vi "AnalyzeBlobs.vi"(9 "Vision Target":enum16{"Pegs", "Gears"}(ring), 10 "Blob Data":T2, 11 "Image In":T3) -> (2 "Target Data":T1, 3 "Image Out":T3)   [LabVIEW 2016]
doc: "Returns if there is a target, and the angle and distance to the target"
uses:
  <vilib>/vision/Image Controls.llb/IMAQ Image.ctl
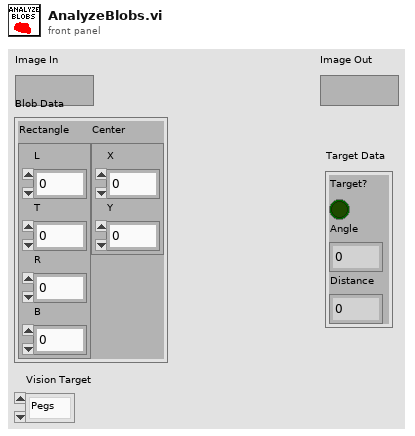
[diagram p1: front panel]
types:
  T1 = cluster{"Target?":bool, "Angle":dbl, "Distance":dbl}
  T2 = cluster{"Rectangle":cluster{"L":dbl, "T":dbl, "R":dbl, "B":dbl}, "Center":cluster{"X":dbl, "Y":dbl}}
  T3 = typedef "IMAQ Image.ctl" = refnum<image>
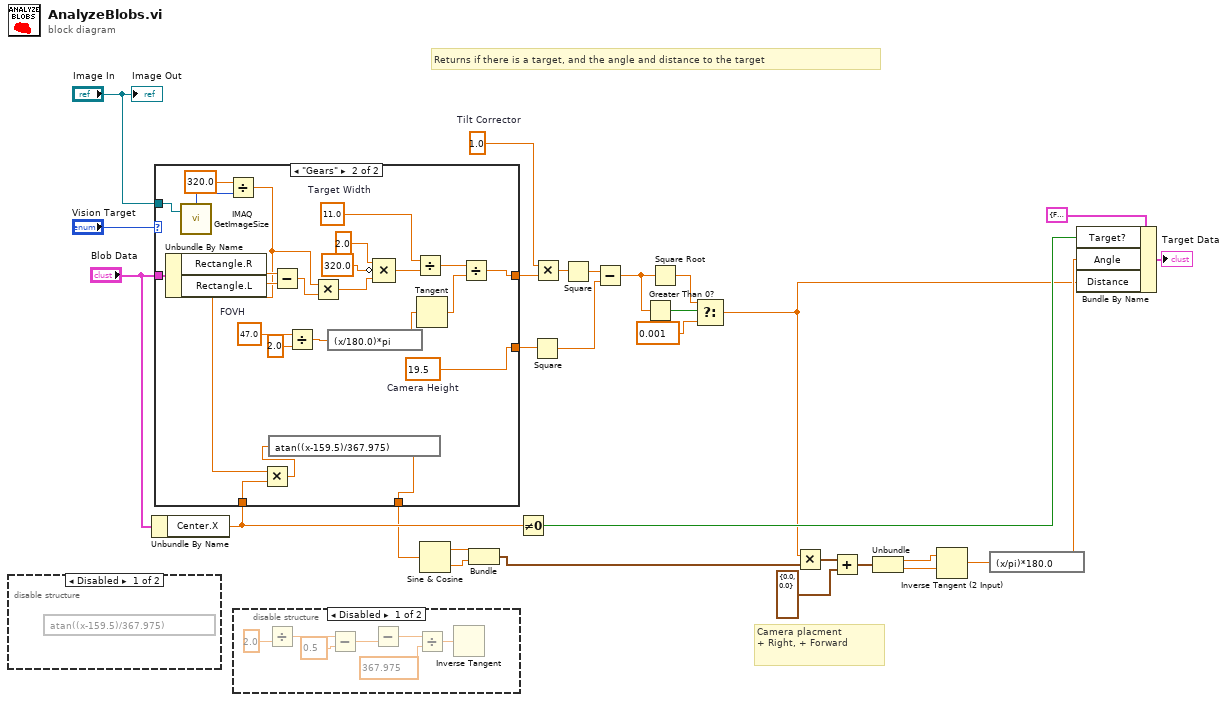
[diagram p0: block diagram]
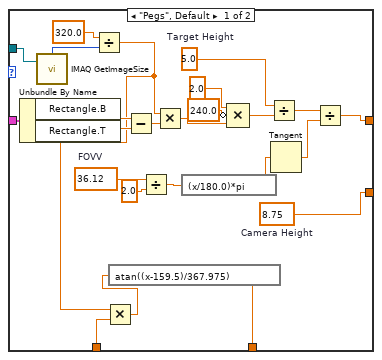
[diagram p4: hidden frame]
diagram:
  w28 = 1.0  # Tilt Corrector
  # "Returns if there is a target, and the angle and distance to the target"
  # "Camera placment\n+ Right, + Forward"
  n1 = disable-structure shown="Disabled" {
    frame Disabled {
      n2 = expression code="atan((x-159.5)/367.975)" ("degrees to radians")() -> ()  [unwired: 1 in, 1 out]
    }
    frame Enabled {
    }
  }
  n3 = Unbundle By Name("Blob Data") -> ("Center.X"=w2:dbl)
  n4 = case shown="\"Gears\"" "Vision Target" {
    tunnel: "Blob Data" -> [w53 w77]
    tunnel: [w44 w70] -> w27
    tunnel: [w43 w69] -> w25
    tunnel: "Image In" -> [w38 w64]
    tunnel: w2 -> [w32 w61]
    tunnel: [w37 w62] -> w1
    frame "Pegs", Default {
      w43 = 8.75  # Camera Height
      w49 = 36.12  # FOVV
      w40 = 5.0  # Target Height
      n5 = Unbundle By Name(w53) -> ("Rectangle.B"=w51:dbl, "Rectangle.T"=w52:dbl)
      n6 = call "IMAQ GetImageSize"("Image"=w38) -> ("X Resolution"=w35:i32)  [unwired: 3 in, 2 out]
      n7 = Divide(x=320.0 ("value"), y=w35) -> (x/y=w31:dbl)
      n8 = Multiply(x=w31, y=w32) -> (x*y=w30:dbl)
      n9 = expression code="atan((x-159.5)/367.975)" ("degrees to radians")(w30) -> (w37:dbl)
      n10 = Subtract(x=w51, y=w52) -> (x-y=w34:dbl)
      n11 = Divide(x=w49, y=2.0) -> (x/y=w47:dbl)
      n12 = Multiply(x=w31, y=w34) -> (x*y=w33:dbl)
      n13 = expression code="(x/180.0)*pi" ("degrees to radians")(w47) -> (w46:dbl)
      n14 = Compound Arithmetic op=MULTIPLY(2.0 ("value"), invert 240.0 ("value"), w33) -> (w41:dbl)
      n15 = Divide(x=w40, y=w41) -> (x/y=w39:dbl)
      n16 = Tangent(1:w46) -> (0:w45:dbl)
      n17 = Divide(x=w39, y=w45) -> (x/y=w44:dbl)
    }
    frame "Gears" {
      w69 = 19.5  # Camera Height
      w74 = 47.0  # FOVH
      w66 = 11.0  # Target Width
      n18 = Unbundle By Name(w77) -> ("Rectangle.R"=w75:dbl, "Rectangle.L"=w76:dbl)
      n19 = call "IMAQ GetImageSize"("Image"=w64) -> ("X Resolution"=w57:i32)  [unwired: 3 in, 2 out]
      n20 = Divide(x=320.0 ("value"), y=w57) -> (x/y=w55:dbl)
      n21 = Multiply(x=w55, y=w61) -> (x*y=w60:dbl)
      n22 = expression code="atan((x-159.5)/367.975)" ("degrees to radians")(w60) -> (w62:dbl)
      n23 = Subtract(x=w75, y=w76) -> (x-y=w56:dbl)
      n24 = Divide(x=w74, y=2.0) -> (x/y=w73:dbl)
      n25 = Multiply(x=w55, y=w56) -> (x*y=w54:dbl)
      n26 = expression code="(x/180.0)*pi" ("degrees to radians")(w73) -> (w72:dbl)
      n27 = Compound Arithmetic op=MULTIPLY(2.0 ("value"), invert 320.0 ("value"), w54) -> (w67:dbl)
      n28 = Divide(x=w66, y=w67) -> (x/y=w65:dbl)
      n29 = Tangent(1:w72) -> (0:w71:dbl)
      n30 = Divide(x=w65, y=w71) -> (x/y=w70:dbl)
    }
  }
  n31 = disable-structure shown="Disabled" {
    frame Disabled {
      n32 = Divide(y=2.0) -> (x/y=w81:dbl)  [unwired: 1 in]
      n33 = Subtract(x=w81, y=0.5) -> (x-y=w79:dbl)
      n34 = Subtract(y=w79) -> (x=w85:dbl, x-y=w78:dbl)
      n35 = Divide(x=w78, y=367.975) -> (x/y=w82:dbl)
      n36 = Inverse Tangent(1:w82) -> ()  [unwired: 1 out]
    }
    frame Enabled {
    }
  }
  n37 = Sine & Cosine(0:w1) -> (1:w18:dbl, 2:w17:dbl)
  n38 = Bundle(w18, w17) -> (w16:cluster{dbl, dbl})  [unwired: 1 in]
  n39 = Not Equal To 0?(x=w2) -> (x != 0?=w19:bool)
  n40 = Square(x=w25) -> (x^2=w23:dbl)
  n41 = Multiply(x=w28, y=w27) -> (x*y=w26:dbl)
  n42 = Square(x=w26) -> (x^2=w24:dbl)
  n43 = Subtract(x=w24, y=w23) -> (x-y=w8:dbl)
  n44 = Greater Than 0?(x=w8) -> (x > 0?=w7:bool)
  n45 = Square Root(x=w8) -> (sqrt(x)=w5:dbl)
  n46 = Select(t=w5, s=w7, f=0.001) -> (s? t:f=w4:dbl)
  n47 = Multiply(x=w4, y=w16) -> (x*y=w15:cluster{dbl, dbl})
  n48 = Add(x=w15, y=cluster{dbl, dbl} {0.0, 0.0}) -> (x+y=w13:cluster{dbl, dbl})
  n49 = Unbundle(w13) -> (w12:dbl, w11:dbl)
  n50 = Inverse Tangent (2 Input)(1:w11, 2:w12) -> (0:w10:dbl)
  n51 = expression code="(x/pi)*180.0" ("radians to degrees")(w10) -> (w9:dbl)
  n52 = Bundle By Name(cluster=T1 {"Target?"=FALSE, "Angle"=0.0, "Distance"=0.0} ("Target Data"), "Target?"=w19, "Angle"=w9, "Distance"=w4) -> (→"Target Data":T1)
  "Image Out" <- "Image In"
